vi "LVFunction_Formatter en gras.vi"(2 "Chaîne":string, 3 "Contrôle chaîne":refnum<vi>) -> (1 "Contrôle chaîne (dup)":refnum<vi>)   [LabVIEW 2020]
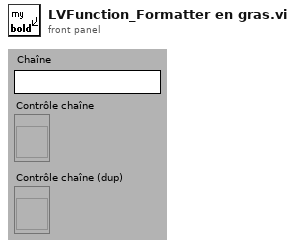
[diagram p1: front panel]
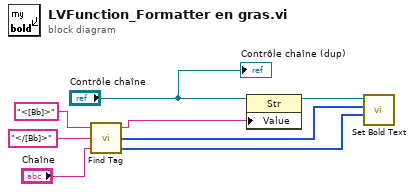
[diagram p0: block diagram]
diagram:
  n1 = call <vilib>:"Find Tag.vi"("string"="Chaîne", "close tag"="</[Bb]>" ("don't translate!"), "open tag"="<[Bb]>" ("don't translate!")) -> ("Length"=w3:i32[], "Start"=w4:i32[], "string out"=w6:string)
  n2 = property on="Property Node" class="Str"(reference="Contrôle chaîne", "Value"=w6) -> (reference out=w5:refnum<vi>)  [unwired: 1 in, 1 out]
  n3 = call <vilib>:"Set Bold Text.vi"("Length"=w3, "Start"=w4, "text"=w5) -> ()  [unwired: 3 in, 1 out]
  "Contrôle chaîne (dup)" <- "Contrôle chaîne"
